vi "Serialize.vi"(8 "error in":errorcluster, 9 "OwningElement in":refnum<k20>, 10 "Document in":refnum<k20>, 11 "DocumentType in":refnum<class "Characteristic.lvclass">) -> (0 "error out":errorcluster, 1 "OwningElement out":refnum<k20>, 2 "Document out":refnum<k20>, 3 "DocumentType out":refnum<class "Characteristic.lvclass">)   [LabVIEW 2021, in "ProligentXMLGenerator.lvlib" / "Characteristic.lvclass"]
uses:
  Characteristic.lvclass
  Characteristic.lvclass/Characteristic.ctl
  Base/DOMSupport/DOMSupport.lvlib
  <vilib>/xml/NI_XML.lvlib
  CustomData/CustomData.lvclass
  <vilib>/xml/Close Reference(Node).vi
  Base/NonEmptyString_434/NonEmptyString_434.lvclass
  C:/Projects/proligent-xml-generator-labview/src/ProligentXMLGenerator/Base/NonEmptyString/NonEmptyString.lvclass
  C:/Projects/proligent-xml-generator-labview/src/ProligentXMLGenerator/Base/String/String.lvclass
  C:/Projects/proligent-xml-generator-labview/src/ProligentXMLGenerator/Base/Attribute/Attribute.lvclass
  C:/Projects/proligent-xml-generator-labview/src/ProligentXMLGenerator/Base/NonEmptyString_434/NonEmptyString_434.lvclass
  Base/String_2000/String_2000.lvclass
  C:/Projects/proligent-xml-generator-labview/src/ProligentXMLGenerator/Base/String_2000/String_2000.lvclass
  Base/String/String.lvclass
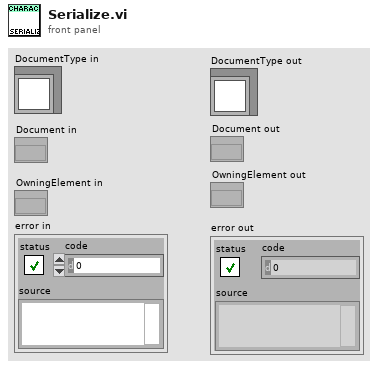
[diagram p1: front panel]
types:
  T1 = typedef "ProligentXMLGenerator.lvlib/Characteristic.lvclass/Data.ctl" = cluster{"Name":string, "CustomData":refnum<class "CustomData.lvclass">, "FullName":refnum<class "NonEmptyString_434.lvclass">, "Value":refnum<class "String_2000.lvclass">}
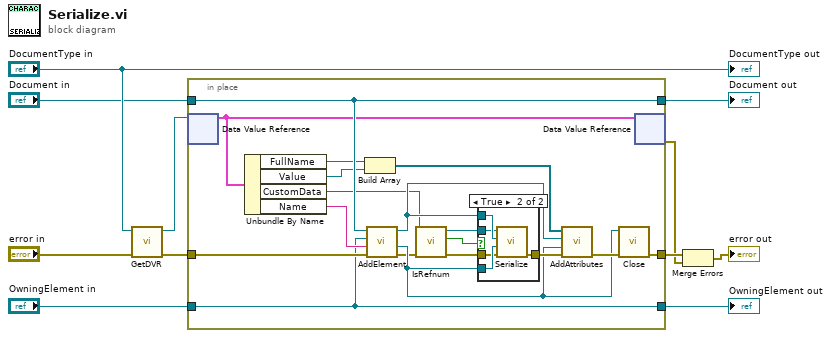
[diagram p0: block diagram]
diagram:
  n1 = call "GetDVR.vi"("error in"="error in", "Document in"="DocumentType in") -> ("error out"=w3:errorcluster, "DVRReference"=w2:refnum<data-value>)  [unwired: 8 in]
  n2 = in-place "In Place Element Structure" {
    in-place-border: [w27] -> w4
    in-place-border: "Document in" -> [w26]
    in-place-border: w3 -> [w29]
    in-place-border: "OwningElement in" -> [w25]
    in-place-border: [w26] -> w6
    in-place-border: [w25] -> w5
    n3 = in-place-dvr #1(w2) -> (w24:T1)  [unwired: 1 out]
    n4 = Unbundle By Name(w24) -> ("FullName"=w20:refnum<class "NonEmptyString_434.lvclass">, "Value"=w12:refnum<class "String_2000.lvclass">, "CustomData"=w15:refnum<class "CustomData.lvclass">, "Name"=w28:string)
    n5 = Build Array(w20, w12) -> (w19:refnum<class "String.lvclass">[])
    n6 = call "AddElement.vi"("error in"=w29, "Name"=w28, "OwningElement in"=w25, "Document in"=w26) -> ("error out"=w18:errorcluster, "NewElement"=w21:refnum<k20>, "Document out"=w16:refnum<k20>)  [unwired: 4 in, 1 out]
    n7 = call "IsRefnum.vi"("error in"=w18, "CustomDataType in"=w15) -> ("error out"=w17:errorcluster, "IsRefnum"=w13:bool, "CustomDataType out"=w14:refnum<class "CustomData.lvclass">)  [unwired: 7 in]
    n8 = case shown="True" w13 {
      tunnel: [w30 w35] -> w23
      tunnel: w21 -> [_ w34]
      tunnel: w17 -> [w30 w33]
      tunnel: w16 -> [_ w32]
      tunnel: w14 -> [_ w31]
      frame False {
      }
      frame True {
        n9 = call "Serialize.vi"("error in"=w33, "OwningElement in"=w34, "Document in"=w32, "CustomDataType in"=w31) -> ("error out"=w35:errorcluster)  [unwired: 4 in, 3 out]
      }
    }
    n10 = call "AddAttributes.vi"("error in"=w23, "OwningElement in"=w21, "Document in"=w16, "Attributes"=w19) -> ("error out"=w22:errorcluster)  [unwired: 5 in, 2 out]
    n11 = call-poly <vilib>:"Close.vi"("error in (no error)"=w22, "node"=w21) -> ("error out"=w27:errorcluster)  [unwired: 7 in]
    n12 = in-place-dvr #1(w24) -> (w1:errorcluster)  [unwired: 1 out]
  }
  "OwningElement out" <- w5
  "Document out" <- w6
  n13 = Merge Errors(w4, w1) -> (→"error out":errorcluster)
  "DocumentType out" <- "DocumentType in"
